vi "Finish.vi"   [LabVIEW 2015]
doc: "This VI is called just before exiting. It is expected to close I/O refnum, save collected data, etc."
uses:
  Robot Global Data.vi
  <vilib>/Rock Robotics/WPI/Utilities/WPI_GetSetVariantRefNum.vi
panel:
  # "FINISH.VI"
types:
  T1 = typedef "WPI_JoystickDevRef.ctl" = cluster{"Device":T2}
  T2 = typedef "WPI_JoystickDeviceEnum.ctl" = enum16{"USB 0", "USB 1", "USB 2", "USB 3", "USB 4", "USB 5"}
  T3 = typedef "WPI_AccelerometerDevRef.ctl" = cluster{"DevStatus":errorcluster, "Scaling":T4, "Analog Channels":T5, "I2C Bus":T7, "SPI Bus":T8, "Accel Range":T9, "ADXL Axes":T10, "Handle":i32, "Device Address":u8, "Accel Type":enum16{"Analog", "ADXL345 I2C", "ADXL345 SPI", "Internal", "ADXL362 SPI"}}
  T4 = typedef "WPI_AccelerometerScaling.ctl" = cluster{"Gain (VoltsPerG)":dbl, "Center Voltage":dbl}
  T5 = typedef "WPI_AccelerometerAnalogChannels.ctl" = cluster{"X-Axis":T6, "Y-Axis":T6, "Z-Axis":T6}
  T6 = typedef "FPGA_AIChannel.ctl" = enum8{"AI 0", "AI 1", "AI 2", "AI 3", "AI MXP 0", "AI MXP 1", "AI MXP 2", "AI MXP 3", "Invalid"}
  T7 = typedef "i2c_bus.ctl" = enum16{"I2C On-Board", "I2C MXP", "Invalid"}
  T8 = typedef "spi_bus.ctl" = enum16{"SPI On-Board, CS0", "SPI On-Board, CS1", "SPI On-Board, CS2", "SPI On-Board, CS3", "SPI MXP", "Invalid"}
  T9 = typedef "ADXL345 Range.ctl" = u8
  T10 = typedef "WPI_AccelerometerADXL345 Axes.ctl" = cluster{"X-Axis":bool, "Y-Axis":bool, "Z-Axis":bool}
  T11 = typedef "WPI_SerialPortRef.ctl" = cluster{"DevStatus":errorcluster, "Serial Port Name":refnum<visa-resource-name>}
  T12 = typedef "WPI_GyroDevRef.ctl" = cluster{"DevStatus":errorcluster, "Analog Channel":T6, "Offset":dbl, "Gain (VoltsPerDegree/Second)":dbl, "Gyro Type":enum16{"Analog", "XRS450"}, "Handle":i32, "SPI Bus":T8, "Device Found":bool, "Sample Rate":dbl, "Calibrate On Open":bool}
  T13 = typedef "WPI_MotorControlDeviceRef.ctl" = cluster{"DeviceStatus":errorcluster, "Type":T14, "PWM":cluster{"PWM Channel":T15, "DeadBand":T16}, "CAN":cluster{"Device Number":u8, "Control Mode":T17, "Semaphore":T18, "Max Vout":dbl, "TalonSRX Control Mode":T19}, "Invert":bool}
  T14 = typedef "WPI_MotorControlType.ctl" = enum16{"PWM", "CAN", "CANTalonSRX"}
  T15 = typedef "FPGA_DIOPWMChannel.ctl" = enum8{"PWM 0", "PWM 1", "PWM 2", "PWM 3", "PWM 4", "PWM 5", "PWM 6", "PWM 7", "PWM 8", "PWM 9", "PWM MXP 0", "PWM MXP 1", "PWM MXP 2", "PWM MXP 3", "PWM MXP 4", "PWM MXP 5", "PWM MXP 6", "PWM MXP 7", "PWM MXP 8", "PWM MXP 9", "Invalid"}
  T16 = typedef "WPI_PWMDeadband.ctl" = cluster{"Name":string, "maxPositivePwm":i32, "minPositivePwm":i32, "centerPwm":i32, "maxNegativePwm":i32, "minNegativePwm":i32, "angularRange":u16}
  T17 = typedef "WPI_CANJaguar_ControlMode.ctl" = enum8{"Percent VBus", "Current", "Speed", "Position", "Voltage"}
  T18 = typedef "Semaphore RefNum" = refnum<k1>
  T19 = typedef "WPI_CANTalonSRX_APIControlMode.ctl" = enum8{"Percent VBus", "Speed", "Position", "Slave", "Unchanged / Invalid", "Voltage Compensation", "Current", "Motion Profile"}
  T20 = typedef "WPI_CompressorDevRef.ctl" = cluster{"DevStatus":errorcluster, "Pneumatics Control Module":u8}
  T21 = typedef "WPI_PotentiometerDevRef.ctl" = cluster{"DevStatus":errorcluster, "Analog Channel":T6, "Invert Output":bool}
  T22 = typedef "WPI_ServoDeviceRef.ctl" = cluster{"DeviceStatus":errorcluster, "PWM Channel":T15, "DeadBand":T16}
  T23 = typedef "WPI_SwitchDevRef.ctl" = cluster{"DevStatus":errorcluster, "DIO Channel":T24, "CntIndex":T25, "Normally Closed":bool}
  T24 = typedef "FPGA_DIOChannel.ctl" = enum8{"DIO 0", "DIO 1", "DIO 2", "DIO 3", "DIO 4", "DIO 5", "DIO 6", "DIO 7", "DIO 8", "DIO 9", "DIO MXP 0", "DIO MXP 1", "DIO MXP 2", "DIO MXP 3", "DIO MXP 4", "DIO MXP 5", "DIO MXP 6", "DIO MXP 7", "DIO MXP 8", "DIO MXP 9", "DIO MXP 10", "DIO MXP 11", "DIO MXP 12", "DIO MXP 13", "DIO MXP 14", "DIO MXP 15", "Invalid"}
  T25 = typedef "FPGA_CounterCtrSystemIndex.ctl" = enum8{"Ctr 0", "Ctr 1", "Ctr 2", "Ctr 3", "Ctr 4", "Ctr 5", "Ctr 6", "Ctr 7", "Invalid"}
  T26 = typedef "WPI_DigitalOutputDevRef.ctl" = cluster{"DIO Channel":T24, "DevStatus":errorcluster}
  T27 = typedef "WPI_I2CDevRef.ctl" = cluster{"DevStatus":errorcluster, "Device Address":u8, "Handle":i32, "I2C Bus":T7}
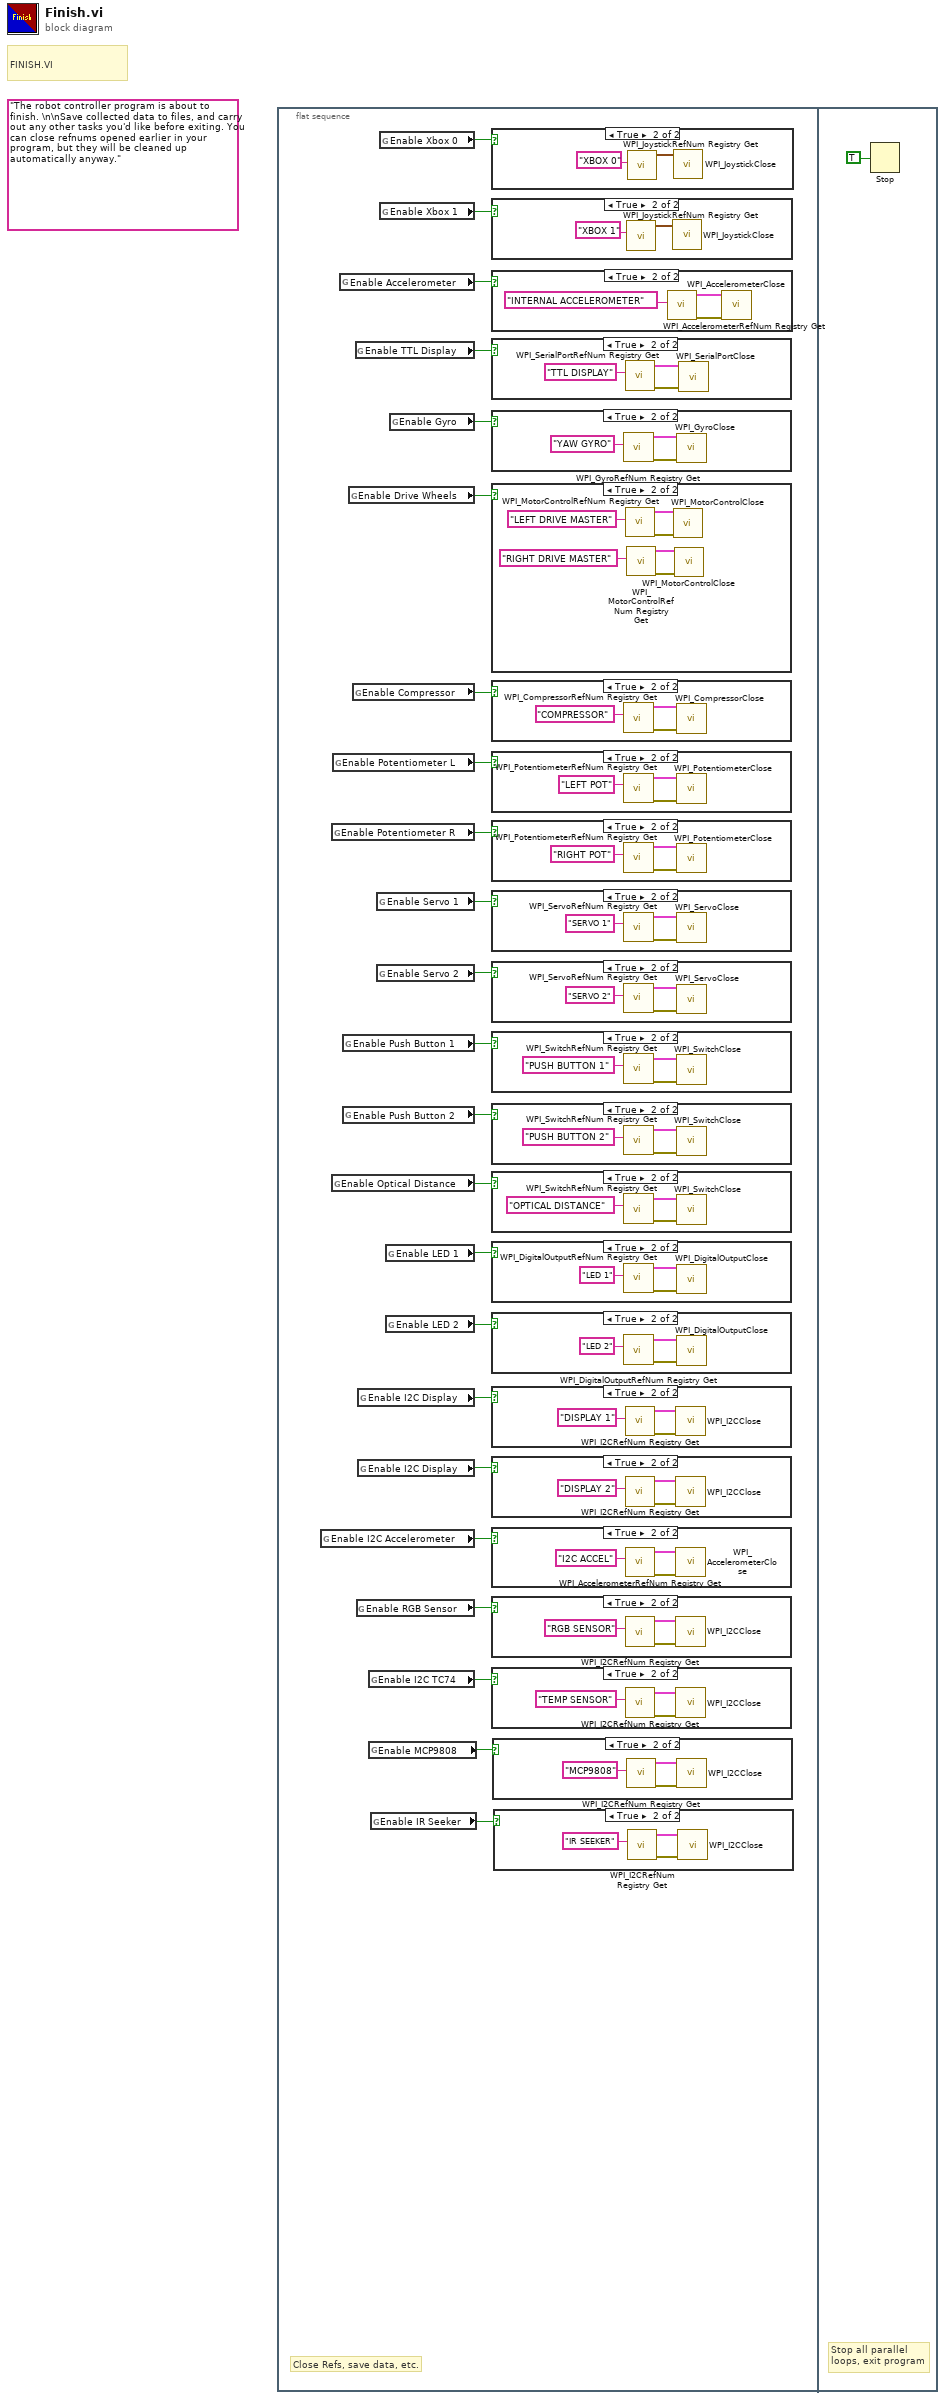
[diagram p0: block diagram]
diagram:
  (unwired) "The robot controller program is about to finish. \n\nSave collected data to files, and carry out any other tasks you'd like before exiting. You can close refnums opened earlier in your program, but they will be cleaned up automatically anyway."
  # "FINISH.VI"
  n1 = flat-sequence {
    frame #0 {
      # "Close Refs, save data, etc."
      n2 = global read "Robot Global Data.vi" "Enable I2C Accelerometer"() -> (w6:bool)
      n3 = global read "Robot Global Data.vi" "Enable Potentiometer R"() -> (w15:bool)
      n4 = global read "Robot Global Data.vi" "Enable Optical Distance"() -> (w10:bool)
      n5 = global read "Robot Global Data.vi" "Enable Potentiometer L"() -> (w16:bool)
      n6 = global read "Robot Global Data.vi" "Enable Accelerometer"() -> (w21:bool)
      n7 = global read "Robot Global Data.vi" "Enable Push Button 1"() -> (w12:bool)
      n8 = global read "Robot Global Data.vi" "Enable Push Button 2"() -> (w11:bool)
      n9 = global read "Robot Global Data.vi" "Enable Drive Wheels"() -> (w18:bool)
      n10 = global read "Robot Global Data.vi" "Enable Compressor"() -> (w17:bool)
      n11 = global read "Robot Global Data.vi" "Enable TTL Display"() -> (w20:bool)
      n12 = global read "Robot Global Data.vi" "Enable RGB Sensor"() -> (w5:bool)
      n13 = global read "Robot Global Data.vi" "Enable I2C Display"() -> (w7:bool)
      n14 = global read "Robot Global Data.vi" "Enable I2C Display"() -> (w4:bool)
      n15 = global read "Robot Global Data.vi" "Enable I2C TC74"() -> (w3:bool)
      n16 = global read "Robot Global Data.vi" "Enable MCP9808"() -> (w2:bool)
      n17 = global read "Robot Global Data.vi" "Enable IR Seeker"() -> (w1:bool)
      n18 = global read "Robot Global Data.vi" "Enable Servo 1"() -> (w14:bool)
      n19 = global read "Robot Global Data.vi" "Enable Servo 2"() -> (w13:bool)
      n20 = global read "Robot Global Data.vi" "Enable Xbox 0"() -> (w23:bool)
      n21 = global read "Robot Global Data.vi" "Enable Xbox 1"() -> (w22:bool)
      n22 = global read "Robot Global Data.vi" "Enable LED 1"() -> (w9:bool)
      n23 = global read "Robot Global Data.vi" "Enable LED 2"() -> (w8:bool)
      n24 = global read "Robot Global Data.vi" "Enable Gyro"() -> (w19:bool)
      n25 = case shown="True" w23 {
        frame False {
        }
        frame True {
          n26 = call <vilib>:"WPI_JoystickRefNum Registry Get.vi"("refnum name"="XBOX 0") -> ("JoystickDevRef"=w92:T1)  [unwired: 1 in, 9 out]
          n27 = call <vilib>:"WPI_JoystickClose.vi"("JoystickDevRef"=w92) -> ()  [unwired: 11 out]
        }
      }
      n28 = case shown="True" w22 {
        frame False {
        }
        frame True {
          n29 = call <vilib>:"WPI_JoystickRefNum Registry Get.vi"("refnum name"="XBOX 1") -> ("JoystickDevRef"=w90:T1)  [unwired: 1 in, 9 out]
          n30 = call <vilib>:"WPI_JoystickClose.vi"("JoystickDevRef"=w90) -> ()  [unwired: 11 out]
        }
      }
      n31 = case shown="True" w21 {
        frame False {
        }
        frame True {
          n32 = call <vilib>:"WPI_AccelerometerRefNum Registry Get.vi"("refnum name"="INTERNAL ACCELEROMETER") -> ("error out"=w87:errorcluster, "AccelerometerDevRef"=w88:T3)  [unwired: 9 in]
          n33 = call <vilib>:"WPI_AccelerometerClose.vi"("error in"=w87, "AccelerometerDevRef"=w88) -> ()  [unwired: 9 in, 1 out]
        }
      }
      n34 = case shown="True" w20 {
        frame False {
        }
        frame True {
          n35 = call <vilib>:"WPI_SerialPortRefNum Registry Get.vi"("refnum name"="TTL DISPLAY") -> ("error out"=w84:errorcluster, "SerialPortRef"=w85:T11)  [unwired: 9 in]
          n36 = call <vilib>:"WPI_SerialPortClose.vi"("error in (no error)"=w84, "SerialPortRef"=w85) -> ()  [unwired: 9 in, 1 out]
        }
      }
      n37 = case shown="True" w19 {
        frame False {
        }
        frame True {
          n38 = call <vilib>:"WPI_GyroRefNum Registry Get.vi"("refnum name"="YAW GYRO") -> ("error out"=w81:errorcluster, "GyroDevRef"=w82:T12)  [unwired: 9 in]
          n39 = call <vilib>:"WPI_GyroClose.vi"("error in"=w81, "GyroDevRef"=w82) -> ()  [unwired: 9 in, 1 out]
        }
      }
      n40 = case shown="True" w18 {
        frame False {
        }
        frame True {
          n41 = call <vilib>:"WPI_MotorControlRefNum Registry Get.vi"("refnum name"="LEFT DRIVE MASTER") -> ("error out"=w78:errorcluster, "MotorControlDevRef"=w79:T13)  [unwired: 9 in]
          n42 = call <vilib>:"WPI_MotorControlRefNum Registry Get.vi"("refnum name"="RIGHT DRIVE MASTER") -> ("error out"=w75:errorcluster, "MotorControlDevRef"=w76:T13)  [unwired: 9 in]
          n43 = call <vilib>:"WPI_MotorControlClose.vi"("error in (no error)"=w78, "MotorControlDevRef"=w79) -> ()  [unwired: 9 in, 1 out]
          n44 = call <vilib>:"WPI_MotorControlClose.vi"("error in (no error)"=w75, "MotorControlDevRef"=w76) -> ()  [unwired: 9 in, 1 out]
        }
      }
      n45 = case shown="True" w17 {
        frame False {
        }
        frame True {
          n46 = call <vilib>:"WPI_CompressorRefNum Registry Get.vi"("refnum name"="COMPRESSOR") -> ("error out"=w72:errorcluster, "CompressorDevRef"=w73:T20)  [unwired: 9 in]
          n47 = call <vilib>:"WPI_CompressorClose.vi"("error in (no error)"=w72, "CompressorDevRef"=w73) -> ()  [unwired: 9 in, 1 out]
        }
      }
      n48 = case shown="True" w16 {
        frame False {
        }
        frame True {
          n49 = call <vilib>:"WPI_PotentiometerRefNum Registry Get.vi"("refnum name"="LEFT POT") -> ("error out"=w69:errorcluster, "PotDevRef"=w70:T21)  [unwired: 9 in]
          n50 = call <vilib>:"WPI_PotentiometerClose.vi"("error in"=w69, "PotDevRef"=w70) -> ()  [unwired: 9 in, 1 out]
        }
      }
      n51 = case shown="True" w15 {
        frame False {
        }
        frame True {
          n52 = call <vilib>:"WPI_PotentiometerRefNum Registry Get.vi"("refnum name"="RIGHT POT") -> ("error out"=w66:errorcluster, "PotDevRef"=w67:T21)  [unwired: 9 in]
          n53 = call <vilib>:"WPI_PotentiometerClose.vi"("error in"=w66, "PotDevRef"=w67) -> ()  [unwired: 9 in, 1 out]
        }
      }
      n54 = case shown="True" w14 {
        frame False {
        }
        frame True {
          n55 = call <vilib>:"WPI_ServoRefNum Registry Get.vi"("refnum name"="SERVO 1") -> ("error out"=w63:errorcluster, "ServoDeviceRef"=w64:T22)  [unwired: 9 in]
          n56 = call <vilib>:"WPI_ServoClose.vi"("error in (no error)"=w63, "ServoDeviceRef"=w64) -> ()  [unwired: 9 in, 1 out]
        }
      }
      n57 = case shown="True" w13 {
        frame False {
        }
        frame True {
          n58 = call <vilib>:"WPI_ServoRefNum Registry Get.vi"("refnum name"="SERVO 2") -> ("error out"=w60:errorcluster, "ServoDeviceRef"=w61:T22)  [unwired: 9 in]
          n59 = call <vilib>:"WPI_ServoClose.vi"("error in (no error)"=w60, "ServoDeviceRef"=w61) -> ()  [unwired: 9 in, 1 out]
        }
      }
      n60 = case shown="True" w12 {
        frame False {
        }
        frame True {
          n61 = call <vilib>:"WPI_SwitchRefNum Registry Get.vi"("refnum name"="PUSH BUTTON 1") -> ("error out"=w57:errorcluster, "SwitchDevRef"=w58:T23)  [unwired: 9 in]
          n62 = call <vilib>:"WPI_SwitchClose.vi"("error in (no error)"=w57, "SwitchDevRef"=w58) -> ()  [unwired: 9 in, 1 out]
        }
      }
      n63 = case shown="True" w11 {
        frame False {
        }
        frame True {
          n64 = call <vilib>:"WPI_SwitchRefNum Registry Get.vi"("refnum name"="PUSH BUTTON 2") -> ("error out"=w54:errorcluster, "SwitchDevRef"=w55:T23)  [unwired: 9 in]
          n65 = call <vilib>:"WPI_SwitchClose.vi"("error in (no error)"=w54, "SwitchDevRef"=w55) -> ()  [unwired: 9 in, 1 out]
        }
      }
      n66 = case shown="True" w10 {
        frame False {
        }
        frame True {
          n67 = call <vilib>:"WPI_SwitchRefNum Registry Get.vi"("refnum name"="OPTICAL DISTANCE") -> ("error out"=w51:errorcluster, "SwitchDevRef"=w52:T23)  [unwired: 9 in]
          n68 = call <vilib>:"WPI_SwitchClose.vi"("error in (no error)"=w51, "SwitchDevRef"=w52) -> ()  [unwired: 9 in, 1 out]
        }
      }
      n69 = case shown="True" w9 {
        frame False {
        }
        frame True {
          n70 = call <vilib>:"WPI_DigitalOutputRefNum Registry Get.vi"("refnum name"="LED 1") -> ("error out"=w49:errorcluster, "DigitalOutputDevRef"=w48:T26)  [unwired: 9 in]
          n71 = call <vilib>:"WPI_DigitalOutputClose.vi"("error in (no error)"=w49, "DigitalOutputDevRef"=w48) -> ()  [unwired: 9 in, 1 out]
        }
      }
      n72 = case shown="True" w8 {
        frame False {
        }
        frame True {
          n73 = call <vilib>:"WPI_DigitalOutputRefNum Registry Get.vi"("refnum name"="LED 2") -> ("error out"=w46:errorcluster, "DigitalOutputDevRef"=w45:T26)  [unwired: 9 in]
          n74 = call <vilib>:"WPI_DigitalOutputClose.vi"("error in (no error)"=w46, "DigitalOutputDevRef"=w45) -> ()  [unwired: 9 in, 1 out]
        }
      }
      n75 = case shown="True" w7 {
        frame False {
        }
        frame True {
          n76 = call <vilib>:"WPI_I2CRefNum Registry Get.vi"("refnum name"="DISPLAY 1") -> ("error out"=w43:errorcluster, "I2CDevRef"=w44:T27)  [unwired: 9 in]
          n77 = call <vilib>:"WPI_I2CClose.vi"("error in (no error)"=w43, "I2CDevRef"=w44) -> ()  [unwired: 9 in, 1 out]
        }
      }
      n78 = case shown="True" w4 {
        frame False {
        }
        frame True {
          n79 = call <vilib>:"WPI_I2CRefNum Registry Get.vi"("refnum name"="DISPLAY 2") -> ("error out"=w34:errorcluster, "I2CDevRef"=w35:T27)  [unwired: 9 in]
          n80 = call <vilib>:"WPI_I2CClose.vi"("error in (no error)"=w34, "I2CDevRef"=w35) -> ()  [unwired: 9 in, 1 out]
        }
      }
      n81 = case shown="True" w6 {
        frame False {
        }
        frame True {
          n82 = call <vilib>:"WPI_AccelerometerRefNum Registry Get.vi"("refnum name"="I2C ACCEL") -> ("error out"=w41:errorcluster, "AccelerometerDevRef"=w39:T3)  [unwired: 9 in]
          n83 = call <vilib>:"WPI_AccelerometerClose.vi"("error in"=w41, "AccelerometerDevRef"=w39) -> ()  [unwired: 9 in, 1 out]
        }
      }
      n84 = case shown="True" w5 {
        frame False {
        }
        frame True {
          n85 = call <vilib>:"WPI_I2CRefNum Registry Get.vi"("refnum name"="RGB SENSOR") -> ("error out"=w38:errorcluster, "I2CDevRef"=w36:T27)  [unwired: 9 in]
          n86 = call <vilib>:"WPI_I2CClose.vi"("error in (no error)"=w38, "I2CDevRef"=w36) -> ()  [unwired: 9 in, 1 out]
        }
      }
      n87 = case shown="True" w3 {
        frame False {
        }
        frame True {
          n88 = call <vilib>:"WPI_I2CRefNum Registry Get.vi"("refnum name"="TEMP SENSOR") -> ("error out"=w32:errorcluster, "I2CDevRef"=w30:T27)  [unwired: 9 in]
          n89 = call <vilib>:"WPI_I2CClose.vi"("error in (no error)"=w32, "I2CDevRef"=w30) -> ()  [unwired: 9 in, 1 out]
        }
      }
      n90 = case shown="True" w2 {
        frame False {
        }
        frame True {
          n91 = call <vilib>:"WPI_I2CRefNum Registry Get.vi"("refnum name"="MCP9808") -> ("error out"=w29:errorcluster, "I2CDevRef"=w27:T27)  [unwired: 9 in]
          n92 = call <vilib>:"WPI_I2CClose.vi"("error in (no error)"=w29, "I2CDevRef"=w27) -> ()  [unwired: 9 in, 1 out]
        }
      }
      n93 = case shown="True" w1 {
        frame False {
        }
        frame True {
          n94 = call <vilib>:"WPI_I2CRefNum Registry Get.vi"("refnum name"="IR SEEKER") -> ("error out"=w26:errorcluster, "I2CDevRef"=w24:T27)  [unwired: 9 in]
          n95 = call <vilib>:"WPI_I2CClose.vi"("error in (no error)"=w26, "I2CDevRef"=w24) -> ()  [unwired: 9 in, 1 out]
        }
      }
    }
    frame #1 {
      # "Stop all parallel\nloops, exit program"
      n96 = Stop(stop? (T)=TRUE ("Quit")) -> ()
    }
  }
